vi "Determine Tilt STATE.vi"(11 "Tilt Data in":T1) -> (3 "Tilt Data out":T1)   [LabVIEW 2020, in "PigeonIMU_SEN.lvlib"]
uses:
  PigeonIMU_SEN.lvlib
  Type Defs/Cluster_Pigeon Tilt Data.ctl
  Shared Code/TypeDefs/ENUM_Tilt State.ctl
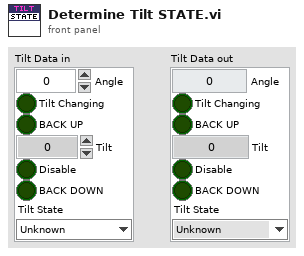
[diagram p1: front panel]
types:
  T1 = typedef "Cluster_Pigeon Tilt Data.ctl" = cluster{"Angle":dbl, "Tilt Changing":bool, "BACK UP":bool, "Tilt":dbl, "Disable":bool, "BACK DOWN":bool, "Tilt State":T2}
  T2 = typedef "ENUM_Tilt State.ctl" = enum16{"Unknown", "Level", "Angle UP from Level", "Level from Angle Up", "Angle Down from Level", "Level from Angle Down"}
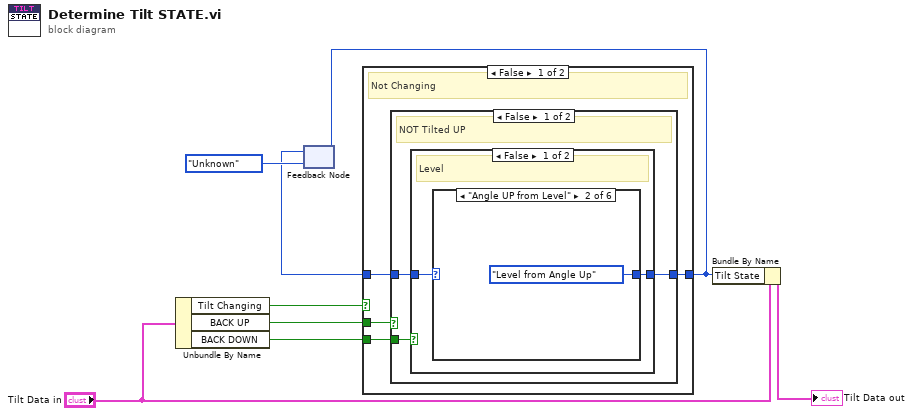
[diagram p0: block diagram]
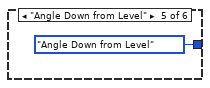
[diagram p5: hidden frame]
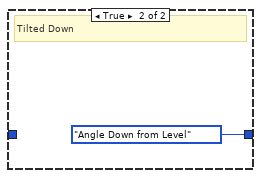
[diagram p7: hidden frame]
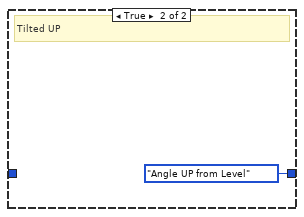
[diagram p8: hidden frame]
diagram:
  n1 = Unbundle By Name("Tilt Data in") -> ("Tilt Changing"=w5:bool, "BACK UP"=w3:bool, "BACK DOWN"=w2:bool)
  n2 = feedback #1(ENUM_Tilt_State."Unknown" ("Tilt State")) -> (w4:T2)
  n3 = case shown="False" w5 {
    tunnel: w4 -> [w10 w26]
    tunnel: [w9 w26] -> w1
    tunnel: w3 -> [w12 _]
    tunnel: w2 -> [w11 _]
    frame False {
      # "Not Changing"
      n4 = case shown="False" w12 {
        tunnel: w11 -> [w15 _]
        tunnel: w10 -> [w14 _]
        tunnel: [w13 ENUM_Tilt_State."Angle UP from Level" ("Tilt State")] -> w9
        frame False {
          # "NOT Tilted UP"
          n5 = case shown="False" w15 {
            tunnel: w14 -> [w17 _]
            tunnel: [w16 ENUM_Tilt_State."Angle Down from Level" ("Tilt State")] -> w13
            frame False {
              # "Level"
              n6 = case shown="\"Angle UP from Level\"" w17 {
                selector: w17 -> [w18 _ w20 w21 _ w23]
                tunnel: [w18 ENUM_Tilt_State."Level from Angle Up" ("Tilt State") w20 w21 ENUM_Tilt_State."Angle Down from Level" ("Tilt State") w23] -> w16
                frame "Unknown" {
                }
                frame "Angle UP from Level" {
                }
                frame "Level from Angle Up" {
                }
                frame "Level from Angle Down" {
                }
                frame "Angle Down from Level" {
                }
                frame "Level" {
                }
              }
            }
            frame True {
              # "Tilted Down"
            }
          }
        }
        frame True {
          # "Tilted UP"
        }
      }
    }
    frame True {
      # "Changing"
    }
  }
  n7 = feedback-in #1(w1) -> ()
  n8 = Bundle By Name(cluster="Tilt Data in", "Tilt State"=w1) -> (→"Tilt Data out":T1)
